vi "Configure IQ Vs Slot Measurement Single List Frequency.vi"(7 "Frequency (0Hz)":dbl format="%#.9p", 8 "error in (no error)":errorcluster, 9 "Index (0)":i32, 10 "Instance (1)":i32=1, 11 "VISA resource name":refnum<visa-resource-name>) -> (0 "error out":errorcluster, 3 "VISA resource name out":refnum<visa-resource-name>)   [LabVIEW 2020, in "Rohde&Schwarz CMXP GPRF.lvlib"]
doc: "Defines the frequency of subsweep <Index>.\n\nAttribute:\nRSCMXPGPRF_ATTR_SET_IQ_VS_SLOT_MEASUREMENT_LIST_STEP_FREQUENCY\n\nRemote-control command:\nCONFigure:GPRF:MEAS<i>:IQVSlot:LIST:FREQuency"
uses:
  <instrlib>/Rohde&Schwarz CMXP GPRF/Rohde&Schwarz CMXP GPRF.lvlib
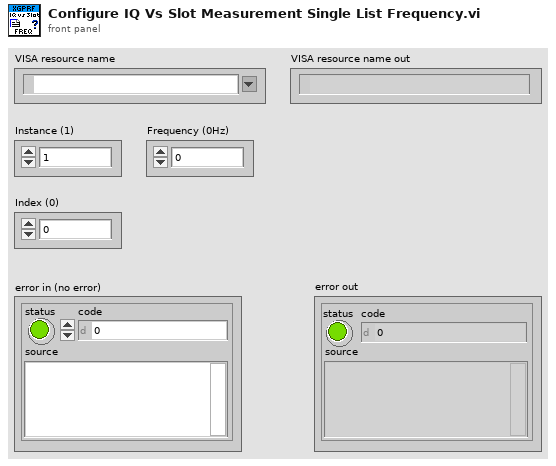
[diagram p1: front panel]
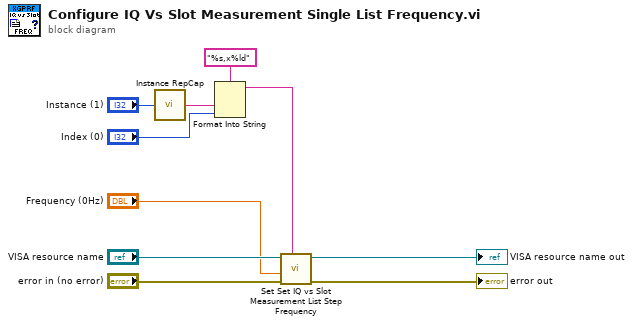
[diagram p0: block diagram]
diagram:
  n1 = call <instrlib>:"Instance RepCap.vi"("Instance in"="Instance (1)") -> ("Instance out"=w6:string)
  n2 = Format Into String(format string="%s,x%ld", w6, "Index (0)") -> (resulting string=w2:string)  [unwired: 2 in, 1 out]
  n3 = call "Set Set IQ vs Slot Measurement List Step Frequency"("Repeated Capabilities"=w2, "error in (no error)"="error in (no error)", "Set IQ vs Slot Measurement List Step Frequency (0.0)"="Frequency (0Hz)", "instrument handle"="VISA resource name") -> ("error out"=→"error out":errorcluster, "instrument handle out"=→"VISA resource name out":refnum<visa-resource-name>)  [unwired: 6 in]
